vi "17- Read data from file and plot it on graph.vi"() -> ()   [LabVIEW 2019]
panel:
  in  "?":bool
  out "Waveform Graph":i32[](graph)
  out "Array of data from file":dbl[](array[numeric])
  out "error out":errorcluster
  in  "file path (use dialog)":path
  # "READ DATA FROM TEXT FILE AND PLOT IT ON GRAPH"
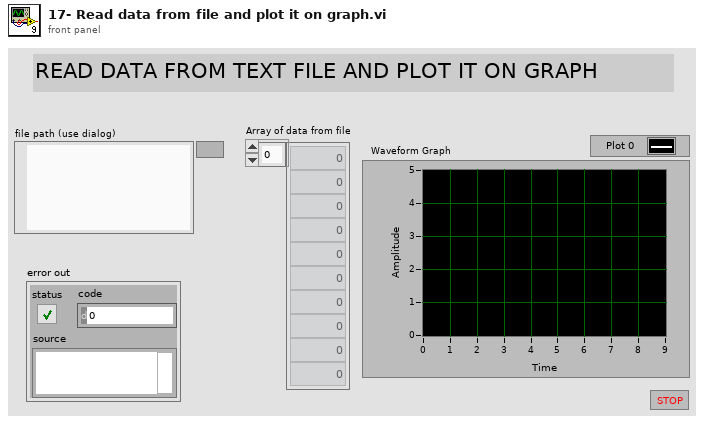
[diagram p1: front panel]
types:
  T1 = enum16{"open", "replace", "create", "open or create", "replace or create", "replace or create with confirmation"}
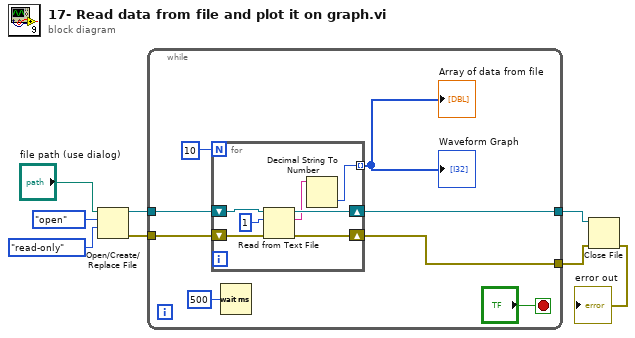
[diagram p0: block diagram]
diagram:
  n1 = Open/Create/Replace File(file path (use dialog)="file path (use dialog)", operation (0:open)=T1."open", access (0:read/write)=enum16{"read/write", "read-only", "write-only"}."read-only") -> (refnum out=w5:refnum<file>, error out=w4:errorcluster)  [unwired: 3 in, 1 out]
  n2 = while {
    tunnel: w5 -> [w12]
    tunnel: w4 -> [w11]
    tunnel: [w10] -> w3
    tunnel: [w9] -> w2
    stop <- "?" stop-if-true
    n3 = for {
      N: 10 -> [_]
      tunnel: [w18] -> w13 mode=indexing
      shift-right: [w22] -> w10
      shift-left: w11 -> [w23]
      shift-right: [w20] -> w9
      shift-left: w12 -> [w21]
      n4 = Read from Text File(file (use dialog)=w21, count=1, error in=w23) -> (refnum out=w20:refnum<file>, text=w19:string, error out=w22:errorcluster)  [unwired: 1 in, 1 out]
      n5 = Decimal String To Number(string=w19) -> (number=w18:i32)  [unwired: 2 in, 1 out]
    }
    "Array of data from file" <- w13
    "Waveform Graph" <- w13
    n6 = Wait (ms)(milliseconds to wait=u32 500) -> ()  [unwired: 1 out]
  }
  n7 = Close File(refnum=w2, error in=w3) -> (error out=→"error out":errorcluster)  [unwired: 1 out]
